vi "080509 FourPMT Detection.vi"() -> ()   [LabVIEW 2009]
doc: "Use this template to measure or generate signals using the DAQ Assistant Express VI and NI-DAQmx. Double click the DAQ Assistant Express VI to launch a configuration wizard which steps you through configuring a measurement or generation.\n\nNote: You must have an NI-DAQmx compatible device installed to use this Express VI. Refer to the DAQ Quick Start Guide for NI-DAQ 7.0 for a list of compatible devices."
uses:
  <vilib>/rvi/interface/nirviOpenFPGA/nirviOpenFPGA.xnode
  FPGA Bitfiles/140824 Sorting FPG~0F_FPGA Target 2_Print drop FPGA--1~2D.lvbitx
  FPGA Four PMTs/Print drop FPGA--140614.vi
  <vilib>/FPGAPlugInAG/Pci-7833r/nirviIntfOpen_PCI-7833R.vi
  <vilib>/rvi/interface/nirviReadWriteControl/nirviReadWriteControl.xnode
  <vilib>/Utility/error.llb/Error Cluster From Error Code.vi
  <vilib>/LabVIEW Targets/FPGA/Rio/nirio_HostInterface/nirio_WriteBig.vi
  <vilib>/rvi/errors/niLvFpgaAdjustHostInterfaceError.vi
  <vilib>/rvi/interface/common/niFpgaNodeNameForErrorReporting.ctl
  <vilib>/rvi/errors/niLvFpgaWhatHappensToTopLevelVI.ctl
  <vilib>/rvi/interface/nirviCloseFPGA/nirviCloseFPGA.xnode
  <vilib>/FPGAPlugInAG/Pci-7833r/nirviIntfClose_PCI-7833R.vi
  <vilib>/rvi/interface/nirviMethod/nirviMethod.xnode
  <vilib>/userDefined/High Color/nirio_resource_hc.ctl
  NiRioSrv.dll
panel:
  out "Host Plot Controls":T1={"refresh"=FALSE, "PMTs for Host"={"Sa"=0, "Sb"=1, "g-factor"=1}, "Peaks"={"# bins"=1000, "min"=0.020751953125, "max"=0.00103759765625}, "Averages"={"# bins"=1000, "max"=0.020751953125, "min"=0.00103759765625}, "Durations"={"# bins"=1000, "max"=20.0, "min"=8.0}, "FP-FPGA"={"# bins"=1000, "max"=20.0, "min"=8.0}, "FP-Host"={"# bins"=1000, "max"=20.0, "min"=8.0}, "Max or Average"=0} {"Max or Average" items=["Peak Max", "Peak Average"]}
  in  "autodetect drops":bool
  out "Sorted":i32
  out "Sort Freq [Hz]":dbl format="%#.1f"
  in  "Peak Detect Maximum [volts]":dbl=10.0
  in  "Maximum duration [ms]":dbl=100.0
  out "#":i32
  out "Iterations":i32
  in  "filename addon":string
  out "#":i32
  in  "baselines":bool=TRUE
  in  "trigger on all":bool
  in  "pause":bool
  in  "base path":path=path "C:/Users/Sean/Desktop"
  in  "all stop":bool
  in  "save timetraces":bool
  in  "save peaks":bool
  in  "Minimum duration [ms]":dbl=0.1
  in  "Peak Detect Minimum [volts]":dbl=0.001
  in  "Primary PMT for Triggering":u8=1
  in  "refresh":bool
  in  "?":T2={"PMT 1"=TRUE, "PMT 2"=TRUE, "PMT 3"=FALSE, "PMT 4"=FALSE}
  out "Drop Freq [Hz]":dbl format="%#.1f"
  out "Detected":i32
  in  "?":T3(tab)
  in  "sort one":bool
  out "Sorting Pulse timetrace":cluster{dbl, dbl, dbl[]}(graph)
  in  "Sorting amplitude [V]":dbl=1.0 min=0.0 max=10.0 step=0.01 format="%_2f"
  in  "Output \nfrequency [Hz]":u32(slide)=30000 step=1 scale=0.0..50000.0
  in  "Burst  cycles":i32(slide)=20 min=1 step=1 scale=0.0..1000.0
  in  "Sorting \ndelay [us]":u32(slide) step=10 scale=0.0..10000.0
  out "detected":i32
  out "sorted":i32
  in  "y":i8(ring)=1 items=["PMT1", "PMT2", "PMT3", "PMT4"]
  in  "x":i8(ring) items=["PMT1", "PMT2", "PMT3", "PMT4"]
  in  "Max or Average":i8(ring) items=["Peak Max", "Peak Average"]
  in  "sort all":bool
  out "?":bool
  in  "Gain 4":sgl(slide)=0.01 min=0.01 max=0.92 step=0.01 scale=0.0..1.0
  in  "Gain 3":sgl(slide)=0.01 min=0.01 max=0.92 step=0.01 scale=0.0..1.0
  in  "Gain 2":sgl(slide)=0.01 min=0.01 max=0.92 step=0.01 scale=0.0..1.0
  in  "Gain 1":sgl(slide)=0.01 min=0.01 max=0.92 step=0.01 scale=0.0..1.0
  in  "autoscale 2":bool=TRUE
  in  "log timetrace":bool
  in  "autoscale":bool
  out "Sorting Timetrace":cluster{dbl, dbl, dbl[][]}(graph)
  in  "bring cursors to center":bool
  out "Peaks":cluster{"Max1":dbl[], dbl[]}[](graph)
  out "HISTOGRAMS  H(durations) vs. durations [ms] 4":cluster{"Axis":dbl[], i32[]}(graph)
  out "HISTOGRAMS  H(peaks) vs peaks [volts] 4":cluster{"Axis":dbl[], i32[]}[](graph)
  in  "#points":i32=1000
  out "working...":bool
  in  "display?":bool=TRUE
  in  "unpack!":bool
  in  "Directory to unpack":path
  out "progress":i32
  out "total":i32
  out "display":cluster{"x*y":dbl, dbl, dbl[][]}(graph)
  in  "extraction duration (s)":dbl=0.1
  out "Time [s]":sgl format="%.1f"
  in  "Acq Rate [Hz]":dbl=40000.0 min=1.0 max=1000000.0 step=1.0 format="%#_12p"
  out "all stop hidden":bool
  out "Vi(t)":cluster{dbl, dbl, dbl[][]}(graph)
  out "peaks data":T4
  out "Baselines":dbl[](array[numeric])
  # "Aquisition  Progress"
  # "Detection Parameters"
  # "Display"
  # "Save Data"
  # "Function Generator"
  # "Pause data collection to increase unpack speed"
  # "I would like to:"
  # "DETECT..."
  # "(1) Select the PMTs to monitor under the \"Display\" panel.\n\n(2) Set PMT power under \"PMT Power\" tab.\n       *Ensure that signal does not rise to 10 V to prevent damaging PMTs.\n       *If program detects PMT saturation they will be automatically powered down.\n\n(3) Specify detection parameters on the left-hand panel.\n       *Drops are identified using only a single PMT signal. You specify which to use with the \"Primary PMT for\n         Triggering\" box in the \"Detection Parameters\" panel on the left.\n\n(4) Specify histogram parameters in the \"Droplet Histograms\" and \"Scatter plot and FP\" tabs.\n\n(5) Select which PMTs to use for scatter plots.\n\n(6) Click the \"Refresh\" button to refresh all the plots.\n\n(7) Make sure that the \"display on\" button is pressed in."
  # "DETECT AND SORT..."
  # "(0) Same as above\n\n(1) Under sorting tab specify sorting criteria.\n       *Primary PMT under Detection Parameters is still used to identify drops.\n\n(2) Sorting pulse allows you to compare detection using PMT inputs and sorting pulse outputs."
  # "Detect based on FLUORESENCE POLARIZATION"
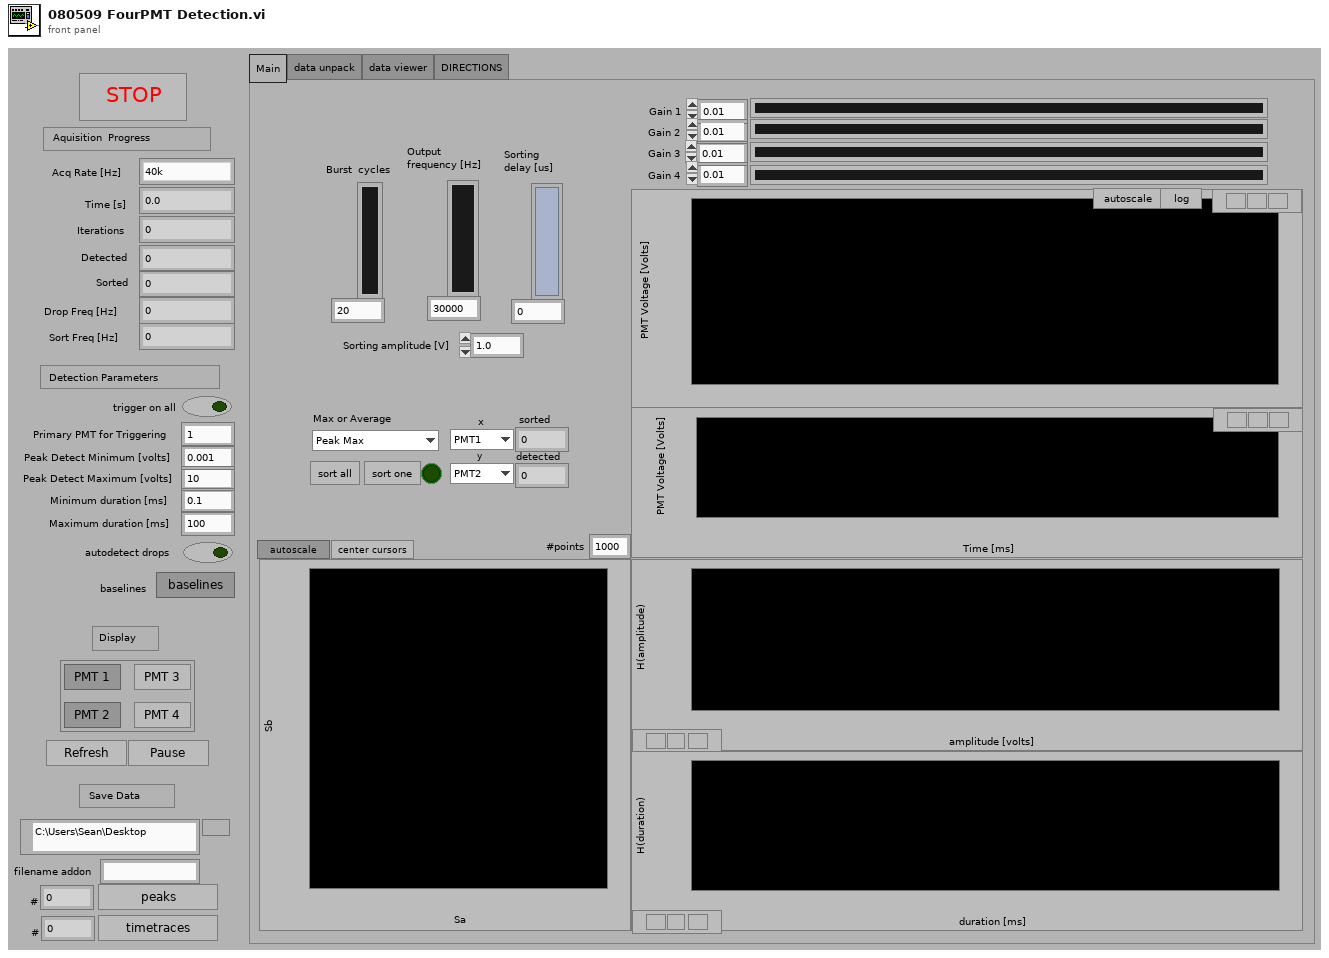
[diagram p1: front panel]
types:
  T1 = cluster{"refresh":bool, "PMTs for Host":cluster{"Sa":i8, "Sb":i8, "g-factor":i32}, "Peaks":cluster{"# bins":i32, "min":dbl, "max":dbl}, "Averages":cluster{"# bins":i32, "max":dbl, "min":dbl}, "Durations":cluster{"# bins":i32, "max":dbl, "min":dbl}, "FP-FPGA":cluster{"# bins":i32, "max":dbl, "min":dbl}, "FP-Host":cluster{"# bins":i32, "max":dbl, "min":dbl}, "Max or Average":i8}
  T2 = cluster{"PMT 1":bool, "PMT 2":bool, "PMT 3":bool, "PMT 4":bool}
  T3 = enum32{"Main", "data unpack", "data viewer", "DIRECTIONS"}
  T4 = cluster{"Maxes":cluster{"Max1":dbl[], "Max2":dbl[], "Max3":dbl[], "Max4":dbl[]}, "Sums":cluster{"Sum1":dbl[], "Sum2":dbl[], "Sum3":dbl[], "Sum4":dbl[]}, "Time in":cluster{"time in":dbl[]}, "Time Out":cluster{"time out":dbl[]}, "FP":cluster{"Sa/Sb or MaxSa":dbl[]}}
  T5 = cluster{"save":bool, dbl, "appended path":path, "refnum":refnum<file>}
  T6 = cluster{"detected":i32, "sorted":dbl, "time [ms]":u32}
  T7 = cluster{"H(durations) out":i32[], "H(average) out":i32[][], "H(peak) out":i32[][], "H(FP) out":i32[], "number of drops detected":i32}
  T8 = typedef "niFpgaNodeNameForErrorReporting.ctl" = enum16{"Open FPGA VI Reference", "Read/Write Control", "Invoke Method: Abort", "Invoke Method: Acknowledge IRQ", "Invoke Method: Download", "Invoke Method: FIFO.Configure", "Invoke Method: FIFO.Read", "Invoke Method: FIFO.Start", "Invoke Method: FIFO.Stop", "Invoke Method: FIFO.Write", "Invoke Method: Reset", "Invoke Method: Run", "Invoke Method: Wait on IRQ", "Close FPGA VI Reference"}
  T9 = typedef "niLvFpgaWhatHappensToTopLevelVI.ctl" = enum16{"top level VI scripted behind XNode", "top level VI inlined behind XNode"}
  T10 = cluster{"Maxes":cluster{"Max1":dbl[], "Max2":dbl[], "Max3":dbl[], "Max4":dbl[]}, "Sums":cluster{"Sum1":dbl[], "Sum2":dbl[], "Sum3":dbl[], "Sum4":dbl[]}, "Time in":cluster{"time in":dbl[]}, "Time Out":cluster{"time out":dbl[]}, "FP":cluster{"Sa/Sb or MaxSa":dbl[]}, "Sort":cluster{"Sort?":dbl[]}}
  T11 = cluster{"refresh":bool, "PMTs for Host":cluster{"Sa":i8, "Sb":i8, "g-factor":i32}, "Peaks":cluster{"# bins":i32, "min":dbl, "max":dbl}, "Averages":cluster{"# bins":i32, "max":dbl, "min":dbl}, "Durations":cluster{"# bins":i32, "max":dbl, "min":dbl}, "FP-FPGA":cluster{"# bins":i32, "max":dbl, "min":dbl}, "FP-Host":cluster{"# bins":i32, "max":dbl, "min":dbl}, "Sort Mode":i8}
  T12 = cluster{"Sorting \ndelay [us]":u32, "Output \nfrequency [Hz]":u32, "Burst  cycles":i32, "Sorting amplitude [V]":dbl}
  T13 = cluster{"Max or Average":i8, "x":i8, "y":i8, "sort all":bool, "Sort below threshold":bool}
  T14 = cluster{"Gain 1":sgl, "Gain 2":sgl, "Gain 3":sgl, "Gain 4":sgl, "Acq Rate [Hz]":dbl, "Primary PMT for Triggering":u8, "Peak Detect Minimum [volts]":dbl, "Peak Detect Maximum [volts]":dbl, "Minimum duration [ms]":dbl, "Maximum duration [ms]":dbl, "Baselines":dbl[], "trigger on all":bool}
  T15 = cluster{"Gain 1":i16, "Gain 2":i16, "Gain 3":i16, "Gain 4":i16, "Acquisition rate [Hz]":u32, "PMT to trigger on":u8, "peak detect minimum":i16, "peak detect maximum":i16, "Minimum Width [ms]":i16, "Maximum Width [ms]":i16, "Baselines":i16[], "trigger on all":bool}
  T16 = cluster{"Sorting Case selection":i8, "Sa":i8, "Sb":i8, "sort?":bool, "Sort below threshold":bool}
  T17 = cluster{"Sorting delay [us]":u32, "Output frequency [Hz]":u32, "Burst  cycles":i32, "Sorting amplitude [V]":i16}
  T18 = cluster{"# bins":i32, "Maximum duration [ms]":dbl, "Minimum duration [ms]":dbl}
  T19 = cluster{"# bins":i32, "Peak Detect Maximum [volts]":dbl, "Peak Detect Minimum [volts]":dbl}
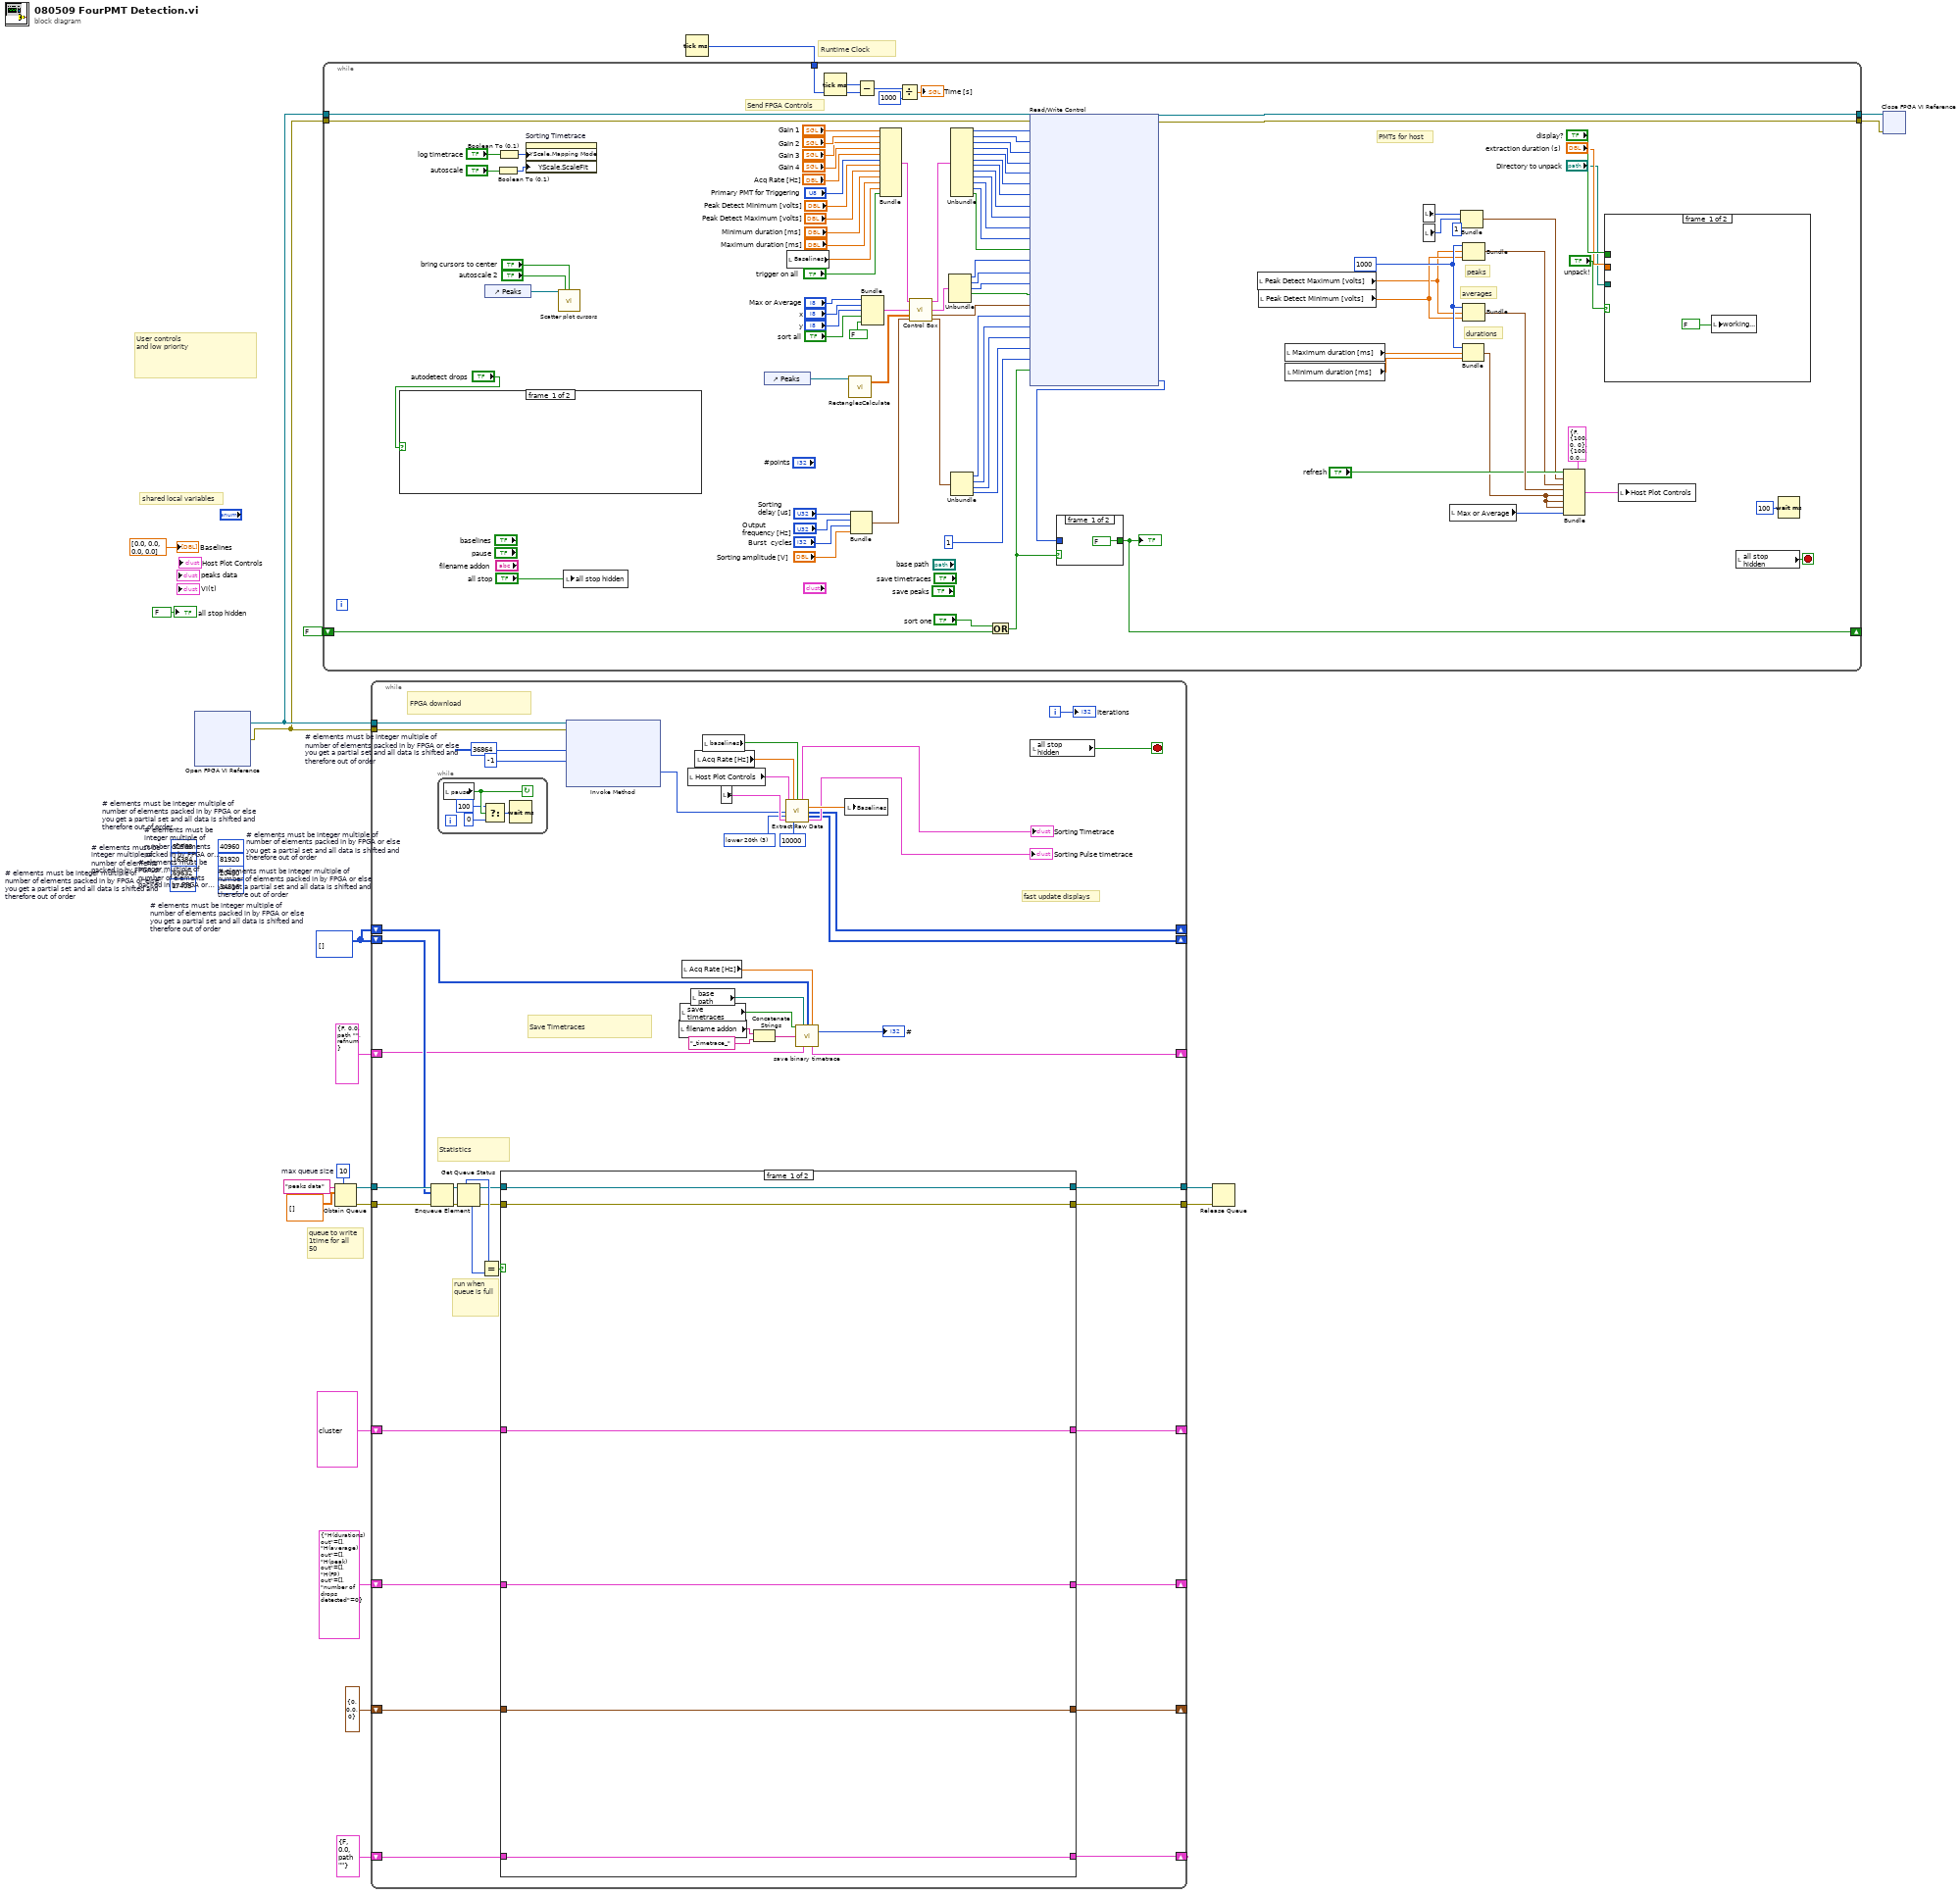
[diagram p0: block diagram]
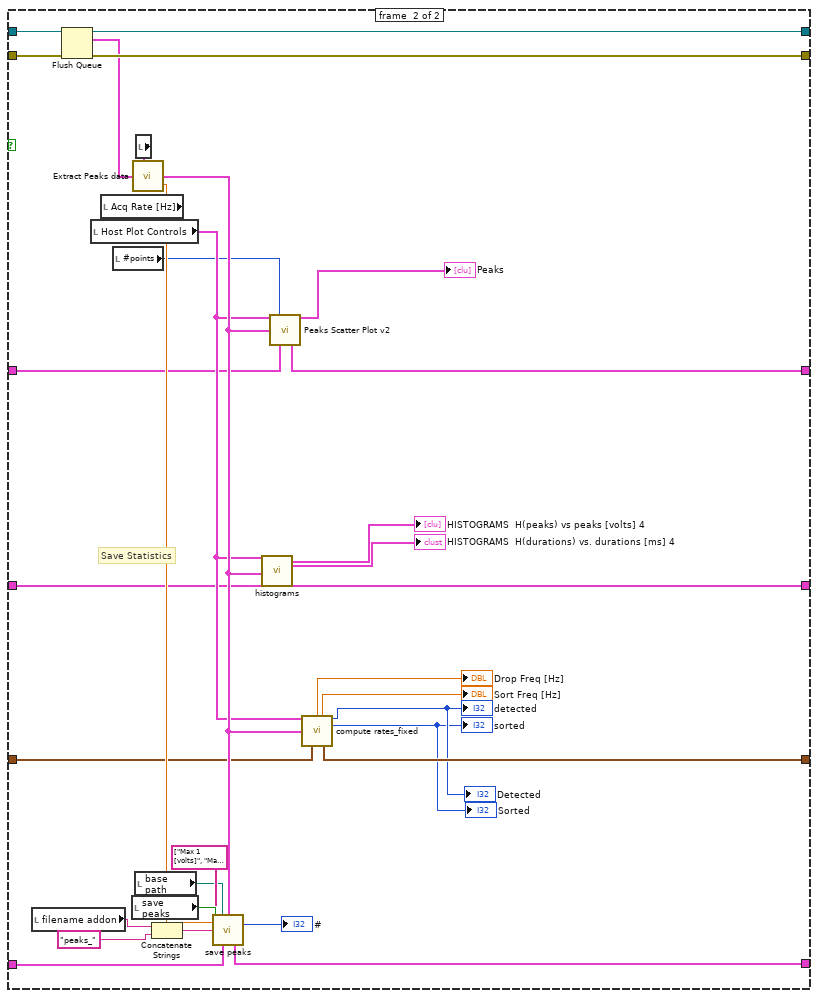
[diagram p2: hidden frame]
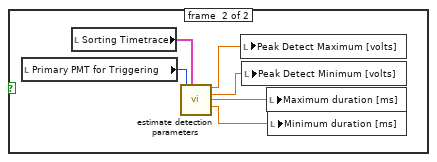
[diagram p3: hidden frame]
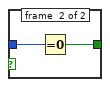
[diagram p4: hidden frame]
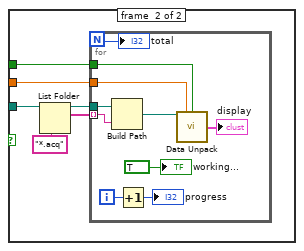
[diagram p5: hidden frame]
diagram:
  w2 = u32[][] [] ("raw peaks data")
  (unwired) u32 17408  # # elements must be integer multiple of number of elements packed in by FPGA or else you get a partial set and all data is shifted and therefore out of order
  (unwired) u32 69632  # # elements must be integer multiple of number of elements packed in by FPGA or else you get a partial set and all data is shifted and therefore out of order
  (unwired) u32 34816  # # elements must be integer multiple of number of elements packed in by FPGA or else you get a partial set and all data is shifted and therefore out of order
  (unwired) u32 40960  # # elements must be integer multiple of number of elements packed in by FPGA or else you get a partial set and all data is shifted and therefore out of order
  (unwired) u32 81920  # # elements must be integer multiple of number of elements packed in by FPGA or else you get a partial set and all data is shifted and therefore out of order
  (unwired) u32 20480  # # elements must be integer multiple of number of elements packed in by FPGA or else you get a partial set and all data is shifted and therefore out of order
  (unwired) u32 16384  # # elements must be integer multiple of number of elements packed in by FPGA or else you get a partial set and all data is shifted and therefore out of order
  (unwired) u32 32768  # # elements must be integer multiple of number of elements packed in by FPGA or else you get a partial set and all data is shifted and therefore out of order
  w14 = 10  # max queue size
  # "queue to write 1time for all 50"
  # "Runtime Clock"
  # "User controls\nand low priority"
  # "shared local variables"
  n1 = xnode "Open FPGA VI Reference"() -> ("FPGA VI Reference Out"=w10:refnum<k20>, "error out"=w9:errorcluster)  [unwired: 2 in]
  n2 = Obtain Queue(max queue size (-1, unlimited)=w14, name (unnamed)="peaks data", element data type=dbl[][] [] ("initialized array")) -> (queue out=w16:refnum<queue>, error out=w17:errorcluster)  [unwired: 2 in, 1 out]
  n3 = while {
    tunnel: w10 -> [w27]
    tunnel: w9 -> [w26]
    tunnel: w16 -> [w62]
    tunnel: [w56] -> w19
    tunnel: [w54] -> w18
    tunnel: w17 -> [w24]
    shift-right: [w49] -> _
    shift-left: T7 {"H(durations) out"=[], "H(average) out"=[], "H(peak) out"=[], "H(FP) out"=[], "number of drops detected"=0} -> [w52]
    shift-right: [w50] -> _
    shift-left: cluster{dbl[], dbl[], dbl[], dbl[]} {array[1000 elements], array[1000 elements], array[1000 elements], array[1000 elements]} -> [w53]
    shift-right: [w47] -> _
    shift-left: cluster{"save":bool, dbl, "appended path":path} {"save"=FALSE, 0.0, "appended path"=path ""} ("shifts out") -> [w48]
    shift-right: [w46] -> _
    shift-left: w2 -> [w45]
    shift-right: [w43] -> _
    shift-left: w2 -> [w35]
    shift-right: [w40] -> _
    shift-left: T5 {"save"=FALSE, 0.0, "appended path"=path "", "refnum"=refnum} ("shifts out") -> [w41]
    shift-right: [w29] -> _
    shift-left: T6 {"detected"=0, "sorted"=0.0, "time [ms]"=0} ("shifts out") -> [w28]
    i -> [w44]
    stop <- w25 stop-if-true
    w22 = 3 items=["median", "noise center", "Minimum", "lower 20th"] ("method")
    w31 = u32 36864  # # elements must be integer multiple of number of elements packed in by FPGA or else you get a partial set and all data is shifted and therefore out of order
    # "Save Timetraces"
    # "run when queue is full"
    # "FPGA download"
    # "Statistics"
    # "fast update displays"
    n4 = Enqueue Element(queue=w62, element=w45, error in (no error)=w24) -> (queue out=w59:refnum<queue>, error out=w58:errorcluster)  [unwired: 1 in, 1 out]
    n5 = while {
      stop <- w111 continue-if-true
      n6 = local read "pause"() -> (w111:bool)
      n7 = Select(t=u32 100 ("milliseconds to wait"), s=w111, f=u32 0) -> (s? t:f=w108:u32)
      n8 = Wait (ms)(milliseconds to wait=w108) -> ()  [unwired: 1 out]
    }
    n9 = Get Queue Status(queue=w59, error in (no error)=w58) -> (queue out=w57:refnum<queue>, max queue size=w60:i32, error out=w55:errorcluster, # elements in queue=w61:i32)  [unwired: 1 in, 4 out]
    n10 = Equal?(x=w60, y=w61) -> (x = y?=w51:bool)
    n11 = case shown="True" w51 {
      tunnel: w57 -> [w75 w104]
      tunnel: [w75 w107] -> w56
      tunnel: w55 -> [w74 w103]
      tunnel: [w74 w106] -> w54
      tunnel: w53 -> [w72 w77]
      tunnel: w52 -> [w73 w83]
      tunnel: [w72 w78] -> w50
      tunnel: [w73 w82] -> w49
      tunnel: w48 -> [w71 w97]
      tunnel: [w71 w96] -> w47
      tunnel: [w70 w86] -> w29
      tunnel: w28 -> [w70 w87]
      frame #0 {
      }
      frame #1 {
        # "Save Statistics"
        n12 = local read "filename addon"() -> (w101:string)
        n13 = Flush Queue(queue=w104, error in (no error)=w103) -> (queue out=w107:refnum<queue>, remaining elements=w102:cluster{"initialized array":dbl[][]}[], error out=w106:errorcluster)
        n14 = local read "Host Plot Controls"() -> (w90:T1)
        n15 = local read "Acq Rate [Hz]"() -> (w93:dbl)
        n16 = local read "#points"() -> (w76:i32)
        n17 = local read "save peaks"() -> (w99:bool)
        n18 = local read "base path"() -> (w94:path)
        n19 = local read item#20() -> (w105:T2)
        n20 = call "Extract Peaks data.vi"("PMTs to monitor:"=w105, "data M1,M2,M3,M4,S1,S2,S3,S4,Tin,Tout,FP"=w102, "Acquisition rate [Hz]"=w93) -> ("peaks data"=w91:T10)  [unwired: 12 in]
        n21 = Concatenate Strings(w101, "peaks_") -> (w98:string)
        n22 = call "save peaks.vi"("save"=w99, "base path"=w94, "peaks data"=w91, "Acq Rate [Hz]"=w93, "column titles"=string[] ["Max 1 [volts]", "Max 2 [volts]", "Max 3 [volts]", "Max 4 [volts]", "ave 1 [volts]", "ave2 [volts]", "ave3", "ave4", "Time inside [ms]", "Time outside [ms]", "Sa/Sb or MaxSa"], "filename"=w98, "shifts in"=w97) -> ("number of files"=→"#":i32, "shifts out"=w96:cluster{"save":bool, dbl, "appended path":path})  [unwired: 5 in, 2 out]
        n23 = call "histograms.vi"("Host Plot Controls"=w90, "peaks data"=w91, 7:w83) -> ("H(peaks) vs peaks [volts]"=→"HISTOGRAMS  H(peaks) vs peaks [volts] 4":cluster{"Axis":dbl[], i32[]}[], "H(durations) vs. durations [ms]"=→"HISTOGRAMS  H(durations) vs. durations [ms] 4":cluster{"Axis":dbl[], i32[]}, 27:w82:T7)  [unwired: 21 in, 1 out]
        n24 = call "Peaks Scatter Plot v2.vi"("Host Plot Controls"=w90, "number to display"=w76, "peaks data"=w91, 12:w77) -> ("scatter"=→"Peaks":cluster{"Max1":dbl[], "Max1":dbl[]}[], 14:w78:cluster{dbl[], dbl[], dbl[], dbl[]})  [unwired: 10 in]
        n25 = call "compute rates_fixed.vi"("Host Plot Controls"=w90, "peaks data"=w91, "shifts in"=w87) -> ("dropfreq"=→"Drop Freq [Hz]":dbl, "sortfreq"=→"Sort Freq [Hz]":dbl, "number detected"=→"Detected" →"detected":i32, "number sorted"=→"sorted" →"Sorted":i32, "shifts out"=w86:T6)  [unwired: 7 in, 1 out]
      }
    }
    n26 = xnode "Invoke Method"("FPGA VI Reference In"=w27, "error in"=w26, "Number of Elements"=w31, "Timeout (ms)"=-1) -> ("Data"=w63:i32[])  [unwired: 3 out]
    n27 = local read "filename addon"() -> (w37:string)
    n28 = local read "save timetraces"() -> (w38:bool)
    n29 = local read "Acq Rate [Hz]"() -> (w32:dbl)
    n30 = local read "Host Plot Controls"() -> (w68:T1)
    n31 = local read "base path"() -> (w42:path)
    n32 = local read "Acq Rate [Hz]"() -> (w69:dbl)
    n33 = local read "baselines"() -> (w64:bool)
    n34 = local read item#20() -> (w66:T2)
    n35 = Concatenate Strings(w37, "_timetrace_") -> (w39:string)
    n36 = call "Extract Raw Data.vi"("Host Plot Controls"=w68, "Acquisition rate [Hz]"=w69, "subtract baseline?"=w64, "FPGA Signal"=w63, "method"=w22, "PMTs to monitor:"=w66, "display length"=10000) -> ("Vi(t)"=→"Sorting Timetrace":cluster{dbl, dbl, dbl[][]}, "Baselines"=w67:dbl[], "raw timetrace data"=w43:u32[][], "raw peaks data"=w46:u32[][], "Sorting Trace"=→"Sorting Pulse timetrace":cluster{dbl, dbl, dbl[]})  [unwired: 1 in, 3 out]
    n37 = call "save binary timetrace.vi"("save"=w38, "base path"=w42, "raw timetrace data"=w35, "Acq Rate [Hz]"=w32, "filename"=w39, "shifts in"=w41) -> ("number of files"=→"#":i32, "shifts out"=w40:T5)  [unwired: 6 in, 2 out]
    n38 = local write "Baselines"(w67) -> ()
    n39 = local read "all stop hidden"() -> (w25:bool)
    "Iterations" <- w44
  }
  n40 = Tick Count (ms)() -> (millisecond timer value=w11:u32)
  n41 = while {
    tunnel: w10 -> [w279]
    tunnel: w9 -> [w278]
    tunnel: w11 -> [w244]
    tunnel: [w221] -> w13
    tunnel: [w220] -> w12
    shift-right: [w207] -> _
    shift-left: FALSE -> [w211]
    stop <- w243 stop-if-true
    w206 = 1000 ("# bins")
    # "PMTs for host"
    # "durations"
    # "peaks"
    # "averages"
    # "Send FPGA Controls"
    n42 = case shown="True" "autodetect drops" {
      frame #0 {
      }
      frame #1 {
        n43 = local read "Primary PMT for Triggering"() -> (w284:u8)
        n44 = local read "Sorting Timetrace"() -> (w285:cluster{dbl, dbl, dbl[][]})
        n45 = call "estimate detection parameters.vi"("PMT for triggering"=w284, "Sorting Timetrace"=w285) -> ("peak max"=w283:dbl, "peak min"=w282:dbl, "max duration"=w281:dbl, "min duration"=w280:dbl)  [unwired: 10 in]
        n46 = local write "Peak Detect Maximum [volts]"(w283) -> ()
        n47 = local write "Peak Detect Minimum [volts]"(w282) -> ()
        n48 = local write "Maximum duration [ms]"(w281) -> ()
        n49 = local write "Minimum duration [ms]"(w280) -> ()
      }
    }
    n50 = control-ref of="Peaks"() -> (w186:refnum<vi>)
    n51 = Boolean To (0,1)(Boolean="autoscale") -> (0, 1=w194:i16)
    n52 = Boolean To (0,1)(Boolean="log timetrace") -> (0, 1=w192:i16)
    n53 = property on="Sorting Timetrace" class="WFGraph (strict)"("YScale.Mapping Mode"=w192, "YScale.ScaleFit"=w194) -> ()  [unwired: 2 in, 2 out]
    n54 = call "Scatter plot cursors.vi"("Peaks"=w186, "autoscale"="autoscale 2", "center cursors"="bring cursors to center") -> ()  [unwired: 13 in]
    n55 = local write "all stop hidden"("all stop") -> ()
    n56 = control-ref of="Peaks"() -> (w201:refnum<vi>)
    n57 = local read "Baselines"() -> (w230:dbl[])
    n58 = Tick Count (ms)() -> (millisecond timer value=w245:u32)
    n59 = call "RectanglesCalculate.vi"("Max"=w201) -> ("Array"=w213:dbl[][])  [unwired: 5 in]
    n60 = Bundle("Sorting \ndelay [us]"="Sorting \ndelay [us]", "Output \nfrequency [Hz]"="Output \nfrequency [Hz]", "Burst  cycles"="Burst  cycles", "Sorting amplitude [V]"="Sorting amplitude [V]") -> (w255:T12)  [unwired: 1 in]
    n61 = Subtract(x=w245, y=w244) -> (x-y=w248:u32)
    n62 = Bundle("Max or Average"="Max or Average", "x"="x", "y"="y", "sort all"="sort all", "Sort below threshold"=FALSE) -> (w251:T13)  [unwired: 1 in]
    n63 = Bundle("Gain 1"="Gain 1", "Gain 2"="Gain 2", "Gain 3"="Gain 3", "Gain 4"="Gain 4", "Acq Rate [Hz]"="Acq Rate [Hz]", "Primary PMT for Triggering"="Primary PMT for Triggering", "Peak Detect Minimum [volts]"="Peak Detect Minimum [volts]", "Peak Detect Maximum [volts]"="Peak Detect Maximum [volts]", "Minimum duration [ms]"="Minimum duration [ms]", "Maximum duration [ms]"="Maximum duration [ms]", "Baselines"=w230, "trigger on all"="trigger on all") -> (w223:T14)  [unwired: 1 in]
    n64 = Divide(x=w248, y=u32 1000) -> (x/y=→"Time [s]":dbl)
    n65 = call "Control Box.vi"("detection controls"=w223, "Sorting parameters"=w251, "Array"=w213, "Function generator"=w255) -> ("detection controls"=w256:T15, "Sorting parameters"=w254:T16, "Array 2"=w212:cluster{"[0]":i32, "[1]":i32, "[2]":i32}[], "Function generator"=w253:T17)  [unwired: 8 in]
    n66 = Unbundle(w254) -> ("Sorting Case selection"=w233:i8, "Sa"=w217:i8, "Sb"=w216:i8, "sort?"=w215:bool)  [unwired: 1 out]
    n67 = Unbundle(w256) -> ("Gain 1"=w270:i16, "Gain 2"=w269:i16, "Gain 3"=w268:i16, "Gain 4"=w267:i16, "Acquisition rate [Hz]"=w266:u32, "PMT to trigger on"=w264:u8, "peak detect minimum"=w265:i16, "peak detect maximum"=w228:i16, "Minimum Width [ms]"=w227:i16, "Maximum Width [ms]"=w226:i16, "Baselines"=w225:i16[], "trigger on all"=w224:bool)
    n68 = Unbundle(w253) -> ("Sorting delay [us]"=w234:u32, "Output frequency [Hz]"=w235:u32, "Burst  cycles"=w236:i32, "Sorting amplitude [V]"=w237:i16)
    n69 = Or(x="sort one", y=w211) -> (x .or. y?=w209:bool)
    n70 = xnode "Read/Write Control"("FPGA VI Reference In"=w279, "error in"=w278, "Gain 1"=w270, "Gain 2"=w269, "Gain 3"=w268, "Gain 4"=w267, "Ticks between acquires (Ticks)"=w266, "PMT to detect drops on"=w264, "Minimum Height"=w265, "Maximum Height"=w228, "Minimum Width"=w227, "Maximum Width"=w226, "Baselines"=w225, "trigger on all"=w224, "Sort Case"=w233, "Sa"=w217, "Sb"=w216, "sort all"=w215, "sorting gates"=w212, "delay [us]"=w234, "1/Frequency  (ticks)"=w235, "Burst  Cycles"=w236, "amplitude"=w237, "window size"=1 ("size"), "sort one"=w209) -> ("FPGA VI Reference Out"=w221:refnum<k20>, "error out"=w220:errorcluster, "N1d"=w208:u32)
    n71 = case shown="True" w209 {
      tunnel: [FALSE w287] -> w207
      tunnel: w208 -> [_ w288]
      frame #0 {
      }
      frame #1 {
        n72 = Equal To 0?(x=w288) -> (x = 0?=w287:bool)
      }
    }
    "?" <- w207
    n73 = local read "Peak Detect Maximum [volts]"() -> (w189:dbl)
    n74 = local read "Peak Detect Minimum [volts]"() -> (w190:dbl)
    n75 = local read "Maximum duration [ms]"() -> (w205:dbl)
    n76 = local read "Minimum duration [ms]"() -> (w204:dbl)
    n77 = local read "x"() -> (w199:i8)
    n78 = local read "y"() -> (w198:i8)
    n79 = local read "Max or Average"() -> (w185:i8)
    n80 = Bundle("x"=w199, "y"=w198, "# bins"=1) -> (w197:cluster{"x":i8, "y":i8, "# bins":i32})  [unwired: 1 in]
    n81 = Bundle("# bins"=w206, "Maximum duration [ms]"=w205, "Minimum duration [ms]"=w204) -> (w202:T18)  [unwired: 1 in]
    n82 = Bundle("# bins"=w206, "Peak Detect Maximum [volts]"=w189, "Peak Detect Minimum [volts]"=w190) -> (w203:T19)  [unwired: 1 in]
    n83 = Bundle("# bins"=w206, "Peak Detect Maximum [volts]"=w189, "Peak Detect Minimum [volts]"=w190) -> (w250:T19)  [unwired: 1 in]
    n84 = Bundle(cluster=T11 {"refresh"=FALSE, "PMTs for Host"={"Sa"=100, "Sb"=0, "g-factor"=0}, "Peaks"={"# bins"=100, "min"=0.01, "max"=0.001}, "Averages"={"# bins"=100, "max"=0.01, "min"=0.001}, "Durations"={"# bins"=100, "max"=40.0, "min"=0.1}, "FP-FPGA"={"# bins"=100, "max"=40.0, "min"=0.1}, "FP-Host"={"# bins"=100, "max"=40.0, "min"=0.1}, "Sort Mode"=0} ("Host Plot Controls"), "refresh"="refresh", "PMTs for Host"=w197, "Peaks"=w203, "Averages"=w250, "Durations"=w202, "FP-FPGA"=w202, "FP-Host"=w202, "Sort Mode"=w185) -> (w184:T11)
    n85 = case shown="True" "unpack!" {
      tunnel: "Directory to unpack" -> [_ w295]
      tunnel: "extraction duration (s)" -> [_ w291]
      tunnel: "display?" -> [_ w290]
      frame #0 {
        n86 = local write "working..."(FALSE ("working...")) -> ()
      }
      frame #1 {
        n87 = List Folder(path=w295, pattern="*.acq") -> (path out=w293:path, filenames=w292:string[])  [unwired: 2 in, 2 out]
        n88 = for {
          N -> [w305]
          tunnel: w293 -> [w304]
          tunnel: w292 -> [w303] mode=indexing
          tunnel: w291 -> [w300]
          tunnel: w290 -> [w299]
          i -> [w298]
          n89 = Build Path(base path=w304, name or relative path=w303) -> (appended path=w302:path)
          n90 = Increment(x=w298) -> (x+1=→"progress":i32)
          n91 = call "Data Unpack.vi"("acquisition file to unpack"=w302, "extraction duration (s)"=w300, "display?"=w299) -> ("display"=→"display":cluster{"y":dbl, dbl, dbl[][]})  [unwired: 12 in]
          "total" <- w305
          "working..." <- TRUE ("working...")
        }
      }
    }
    n92 = local write "Host Plot Controls"(w184) -> ()
    n93 = local read "all stop hidden"() -> (w243:bool)
    n94 = Wait (ms)(milliseconds to wait=u32 100) -> ()  [unwired: 1 out]
  }
  n95 = Release Queue(queue=w19, error in (no error)=w18) -> ()  [unwired: 1 in, 3 out]
  n96 = xnode "Close FPGA VI Reference"("FPGA VI Reference In"=w13, "error in"=w12) -> ()  [unwired: 1 out]
  "Baselines" <- dbl[] [0.0, 0.0, 0.0, 0.0] ("Baselines")
  "all stop hidden" <- FALSE ("all stop hidden")
